vi "pre-suite action.vi"(8 "error in (no error)":errorcluster, 11 "Test Runner.JUnit in":refnum<class "Test Runner.JUnit.lvclass">) -> (0 "error out":errorcluster, 3 "Test Runner.JUnit out":refnum<class "Test Runner.JUnit.lvclass">)   [LabVIEW 2013, in "Test Runner.JUnit.lvclass"]
uses:
  Test Runner.JUnit.lvclass
  classes/Test Runner/Test Runner.lvclass/Test Runner.ctl
  Test Runner.JUnit.lvclass/Test Runner.JUnit.ctl
  classes/Test Runner/Test Runner.lvclass
  classes/Test Report.JUnit/Test Report.JUnit.lvclass
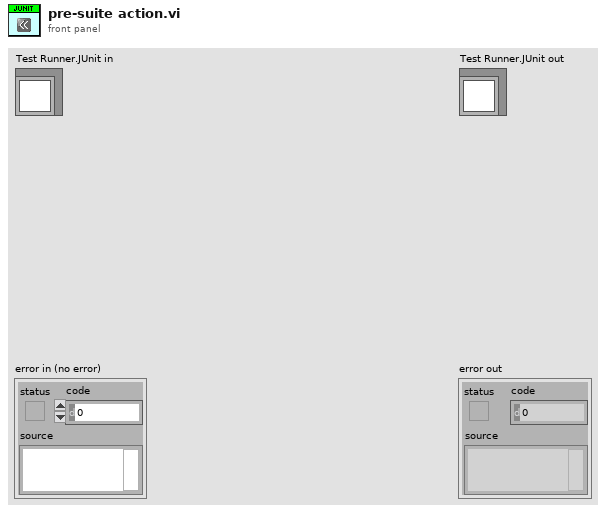
[diagram p1: front panel]
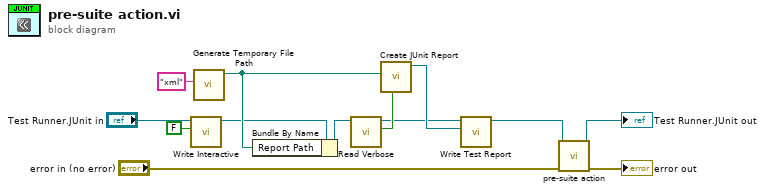
[diagram p0: block diagram]
diagram:
  n1 = call "Write Interactive.vi"("Interactive"=FALSE, "Test Runner in"="Test Runner.JUnit in") -> ("Test Runner out"=w1:refnum<class "Test Runner.JUnit.lvclass">)  [unwired: 9 in]
  n2 = call <vilib>:"Generate Temporary File Path.vi"("Temporary File Extension (tmp)"="xml") -> ("Unique Temporary File Path"=w9:path)  [unwired: 9 in, 1 out]
  n3 = Bundle By Name(cluster=w1, "Report Path"=w9) -> (w4:refnum<class "Test Runner.JUnit.lvclass">)
  n4 = call "Read Verbose.vi"("Test Runner in"=w4) -> ("Verbose"=w6:bool, "Test Runner out"=w5:refnum<class "Test Runner.JUnit.lvclass">)  [unwired: 9 in]
  n5 = call "Create JUnit Report.vi"("Verbose"=w6, "Report Path"=w9) -> ("Test Report.JUnit out"=w11:refnum<class "Test Report.JUnit.lvclass">)  [unwired: 8 in, 1 out]
  n6 = call "Write Test Report.vi"("Test Report"=w11, "Test Runner in"=w5) -> ("Test Runner out"=w7:refnum<class "Test Runner.JUnit.lvclass">)  [unwired: 9 in]
  n7 = call-parent "pre-suite action.vi"("error in (no error)"="error in (no error)", "Test Runner in"=w7) -> ("error out"=→"error out":errorcluster, "Test Runner out"=→"Test Runner.JUnit out":refnum<class "Test Runner.JUnit.lvclass">)  [unwired: 8 in]
